vi "Read Array Ini.vi"(8 "error in (no error)":errorcluster, 10 "Read_key":string[](array[string]), 11 "Section":string) -> (0 "error out":errorcluster, 3 "Result_Value":string[](array[string]))   [LabVIEW 2020]
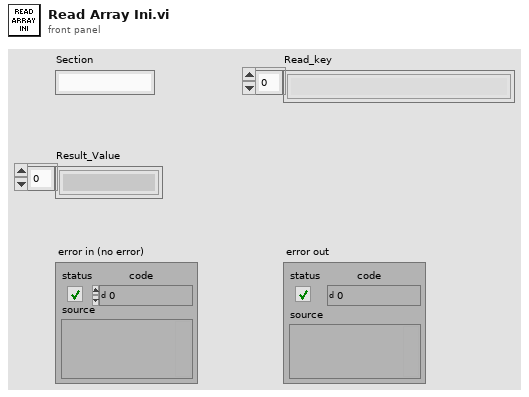
[diagram p1: front panel]
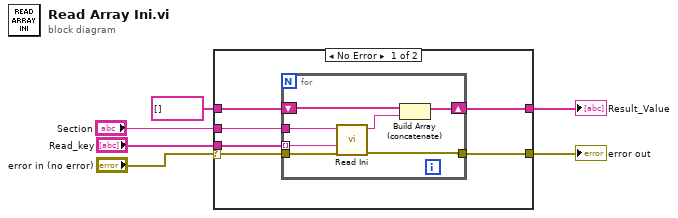
[diagram p0: block diagram]
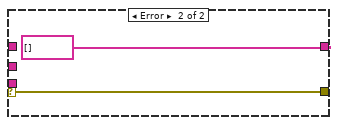
[diagram p2: hidden frame]
diagram:
  n1 = case shown="No Error" "error in (no error)" {
    selector: "error in (no error)" -> [w11 w21]
    tunnel: "Read_key" -> [w12 _]
    tunnel: "Section" -> [w10 _]
    tunnel: [w9 string[] []] -> w3
    tunnel: [w8 w21] -> w2
    tunnel: string[] [] -> [w7 _]
    frame No Error {
      n2 = for {
        tunnel: w12 -> [w18] mode=indexing
        shift-right: [w14] -> w9
        shift-left: w7 -> [w15]
        tunnel: w11 -> [w19]
        tunnel: w10 -> [w17]
        tunnel: [w13] -> w8
        n3 = call "Read Ini.vi"("error in (no error)"=w19, "key"=w18, "section"=w17) -> ("error out"=w13:errorcluster, "value"=w16:string)  [unwired: 7 in]
        n4 = Build Array (concatenate)(w15, w16) -> (w14:string[])
      }
    }
    frame Error {
    }
  }
  "Result_Value" <- w3
  "error out" <- w2
